vi "TissueType.vi"(0 "refnum":refnum<file>, 11 "offset":i32) -> (2 "Tissue Type":T1, 4 "dup refnum":refnum<file>, 6 "organ":i16, 8 "disease type":i16, 10 "disease location":i16, 15 "Blank":string)   [LabVIEW 2022 SP3]
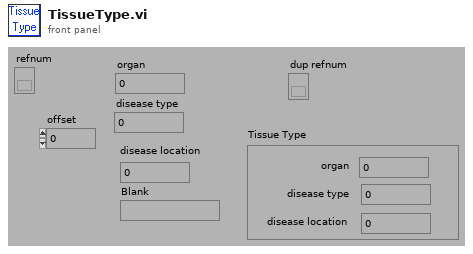
[diagram p1: front panel]
types:
  T1 = cluster{"organ":i16, "disease type":i16, "disease location":i16}
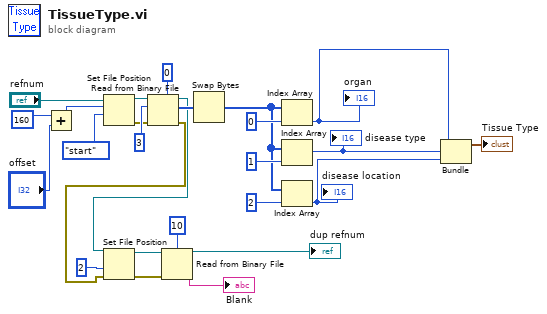
[diagram p0: block diagram]
diagram:
  n1 = Add(x=160 ("pos offset (0)"), y="offset") -> (x+y=w6:i32)
  n2 = Set File Position(offset (in bytes) (0)=w6, refnum="refnum", from (0:start)=enum16{"start", "end", "current"}."start" ("pos mode (0:2)")) -> (refnum out=w5:refnum<file>, error out=w4:errorcluster)  [unwired: 1 in]
  n3 = Read from Binary File(5:i16 0, 8:w4, 10:3 ("count"), 11:w5) -> (0:w1:errorcluster, 2:w17:i16[], 3:w14:refnum<file>)  [unwired: 3 out]
  n4 = Set File Position(refnum=w14, from (0:start)=2, error in=w1) -> (refnum out=w3:refnum<file>, error out=w2:errorcluster)  [unwired: 1 out]
  n5 = Read from Binary File(8:w2, 10:10 ("count"), 11:w3) -> (2:→"Blank":string, 3:→"dup refnum":refnum<file>)  [unwired: 5 out]
  n6 = Swap Bytes(anything=w17) -> (byte swapped=w15:i16[])
  n7 = Index Array(array=w15, index=0) -> (element=w12:i16)
  "organ" <- w12
  n8 = Index Array(array=w15, index=1) -> (element=w11:i16)
  "disease type" <- w11
  n9 = Index Array(array=w15, index=2) -> (element=w10:i16)
  "disease location" <- w10
  n10 = Bundle(w12, w11, w10) -> (→"Tissue Type":cluster{i16, i16, i16})  [unwired: 1 out]
